vi "Renishaw-XL80_SetLambda.vi"(8 "error in (no error)":errorcluster, 10 "Lambda":dbl, 11 "Renishaw-XL80_EMU in":refnum<class "Renishaw-XL80_EMU.lvclass">) -> (0 "error out":errorcluster, 3 "Renishaw-XL80_EMU out":refnum<class "Renishaw-XL80_EMU.lvclass">)   [LabVIEW 2024, in "Renishaw-XL80_EMU.lvclass"]
doc: "Lambda property\nWriting this property will set the wavelength in µm.\n\nDefinition\nHRESULTput_Lambda( [in] double newVal);\nParameters\nnewVal\nSpecifies the wavelength to use (in µm).\n\nComments\nThis property will return with an HRESULT of E_FAIL if the client has not set AutoCompensationMode to AUTO_COMPENSATION_OFF. This warns the client that setting lambda whilst it is being automatically updated is somewhat pointless. Otherwise the property will return an HRESULT of S_OK.\n\n\nSee Also"
uses:
  Renishaw-XL80_EMU.lvclass
  Renishaw-XL80_EMU.lvclass/Renishaw-XL80_EMU.ctl
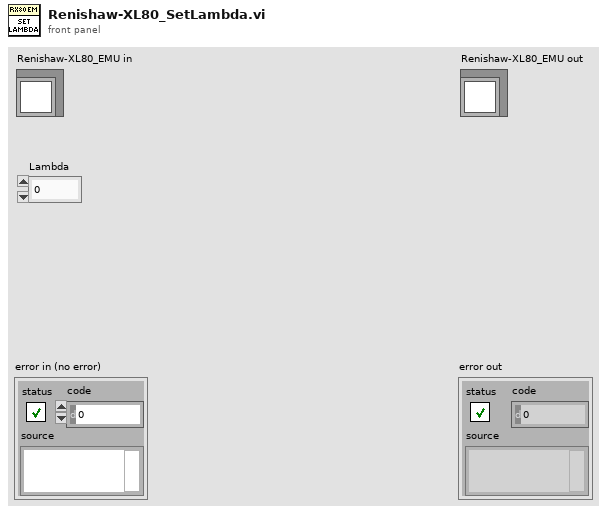
[diagram p1: front panel]
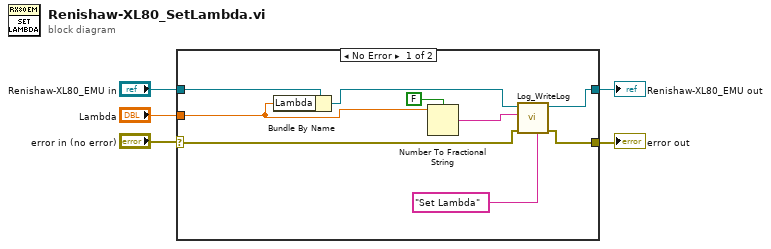
[diagram p0: block diagram]
diagram:
  n1 = case shown="No Error" "error in (no error)" {
    selector: "error in (no error)" -> [w10 w16]
    tunnel: [w11 w16] -> w4
    tunnel: "Renishaw-XL80_EMU in" -> [w14 w15]
    tunnel: [w12 w15] -> w2
    tunnel: "Lambda" -> [w7 _]
    frame No Error {
      n2 = Bundle By Name(cluster=w14, "Lambda"=w7) -> (w13:refnum<class "Renishaw-XL80_EMU.lvclass">)
      n3 = Number To Fractional String(use system decimal point (T)=FALSE, number=w7) -> (F-format string=w6:string)  [unwired: 2 in]
      n4 = call-dynamic "Log_WriteLog.vi"("Additional text"="Set Lambda", "error in (no error)"=w10, "Command"=w6, "Log in"=w13) -> ("error out"=w11:errorcluster, "Log out"=w12:refnum<class "Renishaw-XL80_EMU.lvclass">)  [unwired: 6 in]
    }
    frame Error {
    }
  }
  "error out" <- w4
  "Renishaw-XL80_EMU out" <- w2
